vi "Format to Byte Array to String.vi"(11 "unsigned byte array":u8[](array[numeric]) format="%.0x") -> (3 "String":string)   [LabVIEW 2021, in "Protections.lvlib" / "SMC Protection.lvclass"]
uses:
  SMC Protection.lvclass
  SMC Protection.lvclass/SMC Protection.ctl
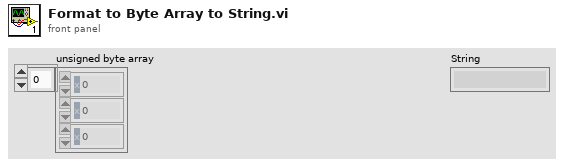
[diagram p1: front panel]
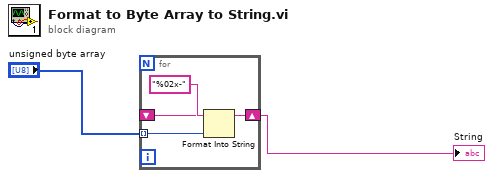
[diagram p0: block diagram]
diagram:
  n1 = for {
    tunnel: "unsigned byte array" -> [w5] mode=indexing
    shift-right: [w4] -> w1
    shift-left: _ -> [w3]
    n2 = Format Into String(format string="%02x-", initial string=w3, w5) -> (resulting string=w4:string)  [unwired: 1 in, 1 out]
  }
  "String" <- w1
